vi "load error enhancer.vi"(8 "error in (no error)":errorcluster, 11 "format string":string) -> (0 "error out":errorcluster)   [LabVIEW 2016, in "SaveLoad.lvlib"]
uses:
  SaveLoad.lvlib
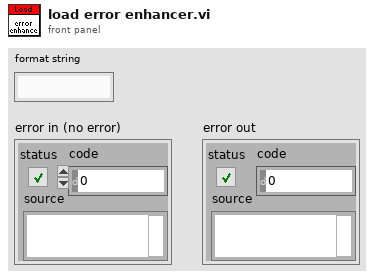
[diagram p1: front panel]
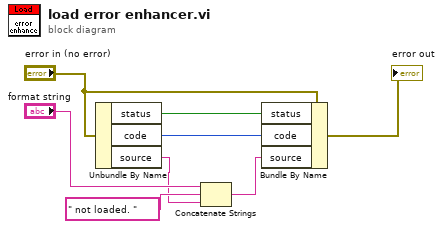
[diagram p0: block diagram]
diagram:
  n1 = Unbundle By Name("error in (no error)") -> ("status"=w1:bool, "code"=w2:i32, "source"=w5:string)
  n2 = Concatenate Strings("format string", " not loaded. " ("string"), w5) -> (w8:string)
  n3 = Bundle By Name(cluster="error in (no error)", "status"=w1, "code"=w2, "source"=w8) -> (→"error out":errorcluster)
